vi "Commit Deposit.vi"(8 "error in (no error)":errorcluster, 10 "User Input":string, 11 "ATM Controller in":refnum<class "ATM Controller.lvclass">) -> (0 "error out":errorcluster, 3 "ATM Controller out":refnum<class "ATM Controller.lvclass">)   [LabVIEW 2020, in "ATM Controller.lvclass"]
uses:
  ATM Controller.lvclass
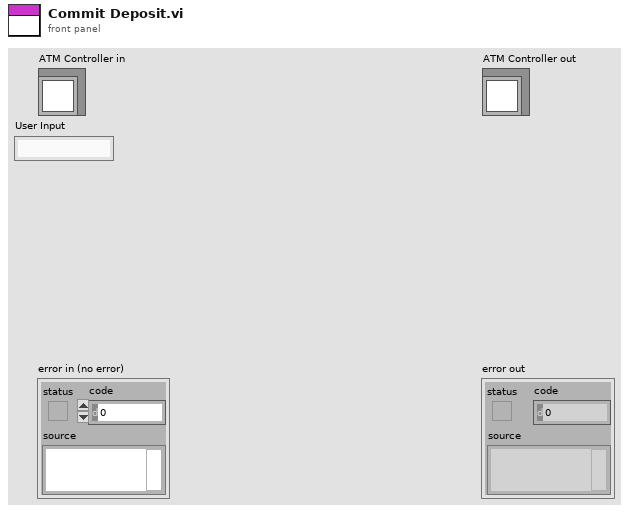
[diagram p1: front panel]
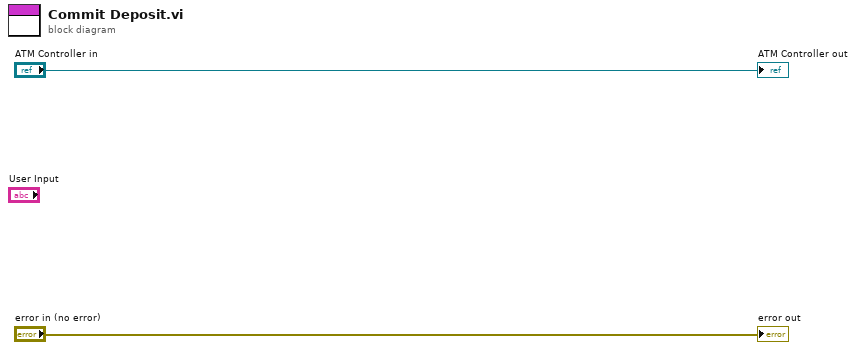
[diagram p0: block diagram]
diagram:
  "error out" <- "error in (no error)"
  "ATM Controller out" <- "ATM Controller in"
